vi "max30102Chart_Plot_step0.vi"() -> ()   [LabVIEW 2014]
doc: "Use this template to build a producer/consumer design pattern. Use this template when you need to execute a process, such as data analysis, when a data source, such as a triggered acquisition, produces data at an uneven rate and you need to execute the process when the data becomes available.\n------------------------------------\nAuther: Koji Ohashi\nCopyright (c) 2020 Japan LabVIEW Users Group, Volunteer members.\nThis VI is released under the MIT License.\nhttp://opensource.org/licenses/mit-license.php\n------------------------------------"
uses:
  <vilib>/Instr/_visa.llb/VISA Configure Serial Port (Instr).vi
panel:
  out "Waveform Chart":i32(graph)
  in  "Read Count":u32=1000
  in  "Termination Character":u8=10 format="%.0x"
  in  "VISA resource name":refnum<visa-resource-name>="COM1"
  in  "Serial Settings":T1={"baud rate"=9600, "data bits"=8, "parity"=enum."None", "stop bits"=10, "flow control"=0} {"flow control" items=["None"=0, "XON/XOFF"=1, "RTS/CTS"=2, "DTR/DSR"=4]; "stop bits" items=["1.0"=10, "1.5"=15, "2.0"=20]; "data bits" min=5 max=8 step=1; "baud rate" items=["75"=75, "110"=110, "134"=134, "150"=150, "300"=300, "600"=600, "1200"=1200, "1800"=1800, "2400"=2400, "4800"=4800, "7200"=7200, "9600"=9600, "14400"=14400, "19200"=19200, "28800"=28800, "38400"=38400, "56000"=56000, "57600"=57600, "115200"=115200, "128000"=128000, "230400"=230400]}
  in  "End Read on Termination Character?":bool=TRUE
  in  "stop":bool
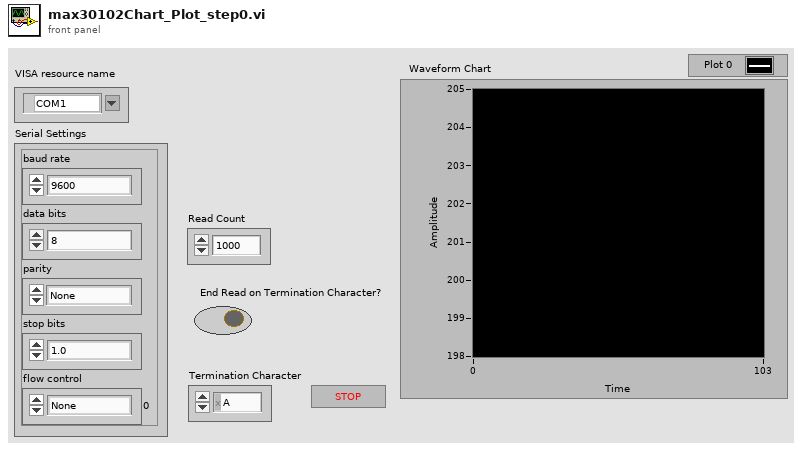
[diagram p1: front panel]
types:
  T1 = cluster{"baud rate":u32, "data bits":u16, "parity":enum16{"None", "Odd", "Even", "Mark", "Space"}, "stop bits":u16, "flow control":u16}
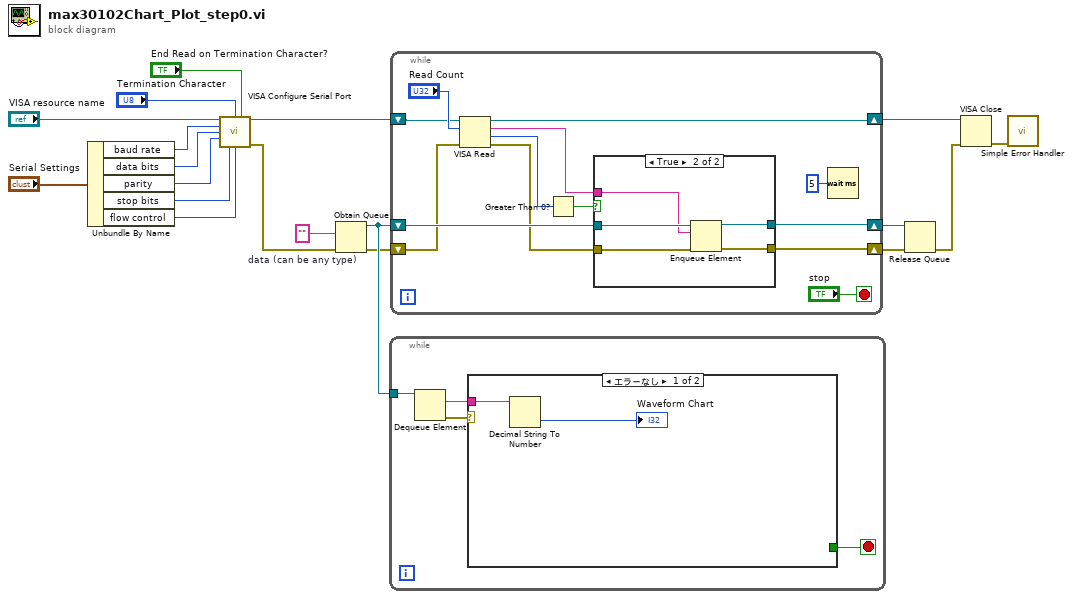
[diagram p0: block diagram]
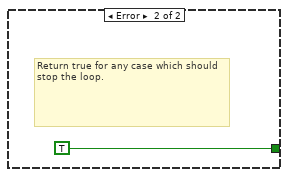
[diagram p2: hidden frame]
diagram:
  w15 = ""  # data (can be any type)
  n1 = Unbundle By Name("Serial Settings") -> ("baud rate"=w10:u32, "data bits"=w11:u16, "parity"=w12:enum16{"None", "Odd", "Even", "Mark", "Space"}, "stop bits"=w13:u16, "flow control"=w7:u16)
  n2 = call-poly "VISA Configure Serial Port"("VISA resource name"="VISA resource name", "termination char\n(0xA = '\\n' = LF)"="Termination Character", "Enable Termination\nChar (T)"="End Read on Termination Character?", "baud rate (9600)"=w10, "data bits (8)"=w11, "parity (0:none)"=w12, "stop bits (10: 1 bit)"=w13, "flow control (0:none)"=w7) -> ("VISA resource name out"=w5:refnum<visa-resource-name>, "error out"=w2:errorcluster)  [unwired: 2 in, 4 out]
  n3 = Obtain Queue(element data type=w15, error in (no error)=w2) -> (queue out=w19:refnum<queue>, error out=w18:errorcluster)  [unwired: 3 in, 1 out]
  n4 = while {
    tunnel: w19 -> [w23]
    stop <- w20 stop-if-true
    n5 = Dequeue Element(queue=w23) -> (element=w21:string, error out=w22:errorcluster)  [unwired: 2 in, 2 out]
    n6 = case shown="エラーなし" w22 {
      tunnel: w21 -> [w25 _]
      tunnel: [_ TRUE] -> w20
      frame No Error {
        n7 = Decimal String To Number(string=w25) -> (number=→"Waveform Chart":i32)  [unwired: 2 in, 1 out]
      }
      frame Error {
        # "Return true for any case which should stop the loop."
      }
    }
  }
  n8 = while {
    shift-right: [w36] -> w16
    shift-left: w18 -> [w29]
    shift-right: [w37] -> w17
    shift-left: w19 -> [w38]
    shift-right: [w33] -> w3
    shift-left: w5 -> [w27]
    stop <- "stop" stop-if-true
    n9 = VISA Read(VISA resource name=w27, byte count="Read Count", error in (no error)=w29) -> (VISA resource name out=w33:refnum<visa-resource-name>, read buffer=w30:string, return count=w32:u32, error out=w28:errorcluster)
    n10 = Greater Than 0?(x=w32) -> (x > 0?=w31:bool)
    n11 = case shown="TRUE" w31 {
      tunnel: w38 -> [w41 w46]
      tunnel: [w41 w45] -> w37
      tunnel: w28 -> [w40 w44]
      tunnel: [w40 w43] -> w36
      tunnel: w30 -> [_ w42]
      frame False {
      }
      frame True {
        n12 = Enqueue Element(queue=w46, element=w42, error in (no error)=w44) -> (queue out=w45:refnum<queue>, error out=w43:errorcluster)  [unwired: 1 in, 1 out]
      }
    }
    n13 = Wait (ms)(milliseconds to wait=u32 5) -> ()  [unwired: 1 out]
  }
  n14 = Release Queue(queue=w17, error in (no error)=w16) -> (error out=w1:errorcluster)  [unwired: 1 in, 2 out]
  n15 = VISA Close(VISA resource name=w3, error in (no error)=w1) -> (error out=w4:errorcluster)
  n16 = call <vilib>:"Simple Error Handler.vi"("error in (no error)"=w4) -> ()  [unwired: 1 in, 8 out]
